vi "ElevatorBrake.vi"(5 "Elevator Manual Mode":bool, 7 "Manual Movement":dbl, 9 "Elevator State In":string, 10 "Elevator Power In":dbl, 11 "Elevator Error":dbl) -> (1 "Elevator State Out":string, 2 "Elevator Power Out":dbl)   [LabVIEW 2018]
uses:
  Inputs_DriverStation.vi
  SensorReadings.vi
  RobotStates.vi
panel:
  in  "Brake Pressure Threshold (PSI)":dbl=30.0
  in  "Hysteresis Threshold (ms)":u32=500
  in  "Time in Error Band (ms)":u32=1000
  in  "Error Band (in)":dbl=20.0
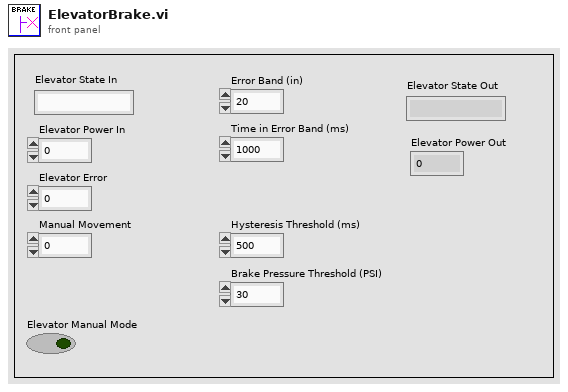
[diagram p1: front panel]
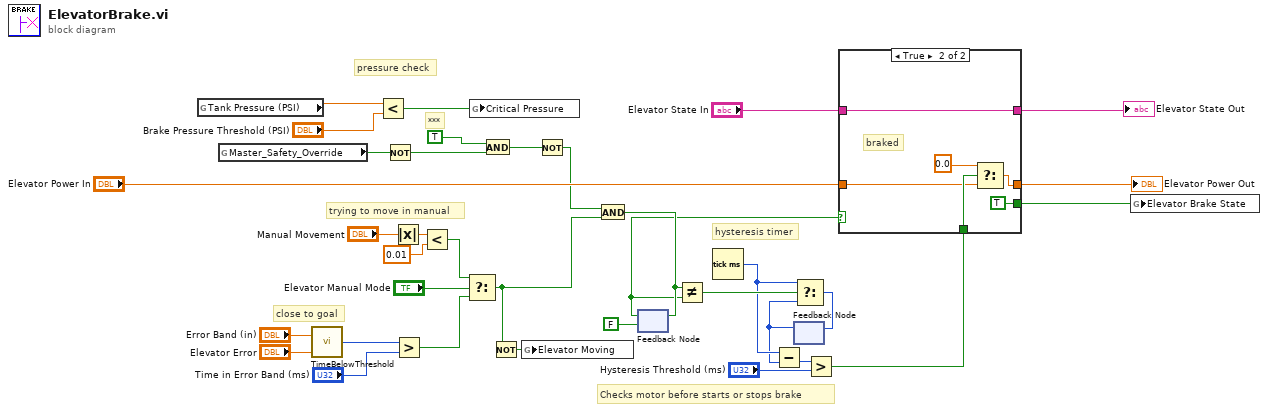
[diagram p0: block diagram]
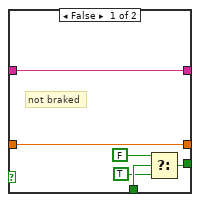
[diagram p2: hidden frame]
diagram:
  # "***"
  # "Checks motor before starts or stops brake"
  # "hysteresis timer"
  # "pressure check"
  # "trying to move in manual"
  # "close to goal"
  n1 = global read "SensorReadings.vi" "Tank Pressure (PSI)"() -> (w7:dbl)
  n2 = global read "Inputs_DriverStation.vi" "Master_Safety_Override"() -> (w23:bool)
  n3 = call "TimeBelowThreshold.vi"("Current Value"="Elevator Error", "Threshold"="Error Band (in)") -> ("Time Below"=w33:u32)  [unwired: 3 in]
  n4 = Less?(x=w7, y="Brake Pressure Threshold (PSI)") -> (x < y?=w6:bool)
  n5 = Not(x=w23) -> (.not. x?=w22:bool)
  n6 = Absolute Value(x="Manual Movement") -> (abs(x)=w30:dbl)
  n7 = Greater?(x=w33, y="Time in Error Band (ms)") -> (0:w28:bool)
  n8 = Less?(x=w30, y=0.01) -> (x < y?=w26:bool)
  n9 = Select(t=w26, s="Elevator Manual Mode", f=w28) -> (s? t:f=w4:bool)
  n10 = global write "SensorReadings.vi" "Critical Pressure"(w6) -> ()
  n11 = And(x=TRUE, y=w22) -> (x .and. y?=w21:bool)
  n12 = Not(x=w4) -> (.not. x?=w3:bool)
  n13 = global write "RobotStates.vi" "Elevator Moving"(w3) -> ()
  n14 = Not(x=w21) -> (.not. x?=w20:bool)
  n15 = And(x=w20, y=w4) -> (x .and. y?=w18:bool)
  n16 = feedback-in #1(w18) -> ()
  n17 = feedback #1(FALSE) -> (w2:bool)
  n18 = Not Equal?(x=w18, y=w2) -> (x != y?=w16:bool)
  n19 = Tick Count (ms)() -> (millisecond timer value=w14:u32)
  n20 = feedback #2() -> (w13:u32)  [unwired: 1 in]
  n21 = Subtract(x=w14, y=w13) -> (x-y=w15:u32)
  n22 = Select(t=w14, s=w16, f=w13) -> (s? t:f=w17:u32)
  n23 = feedback-in #2(w17) -> ()
  n24 = Greater?(x=w15, y="Hysteresis Threshold (ms)") -> (0:w8:bool)
  n25 = case shown="True" w2 {
    tunnel: "Elevator Power In" -> [w41 w42]
    tunnel: [w41 w45] -> w10
    tunnel: [w36 TRUE] -> w11
    tunnel: "Elevator State In" -> [w40 w46]
    tunnel: [w40 w46] -> w9
    tunnel: w8 -> [w39 w43]
    frame False {
      # "not braked"
      n26 = Select(t=FALSE, s=w39, f=TRUE) -> (s? t:f=w36:bool)
    }
    frame True {
      # "braked"
      n27 = Select(t=0.0 ("Elevator Power In"), s=w43, f=w42) -> (s? t:f=w45:dbl)
    }
  }
  "Elevator Power Out" <- w10
  "Elevator State Out" <- w9
  n28 = global write "RobotStates.vi" "Elevator Brake State"(w11) -> ()
